vi "Test one or two lift motors.vi"(10 "Direction 2":enum16{"Stop", "Up", "Down"}(ring), 11 "Direction":enum16{"Stop", "Up", "Down"}(ring)) -> ()   [LabVIEW 2014]
uses:
  <vilib>/Rock Robotics/SystemInterfaces/DIO/FPGA_DIOPWMChannel.ctl
  <vilib>/Rock Robotics/WPI/MotorControl/WPI_MotorControlOpen Talon.vi
panel:
  in  "Mode 2":enum8{"Start", "Run", "Finish"}(ring)
  in  "Down Speed 2":dbl=-0.2 format="%#_13g"
  in  "Up Speed 2":dbl=0.3 format="%#_13g"
  in  "Motor one or two":bool
  in  "Mode":enum8{"Start", "Run", "Finish"}(ring)
  in  "Down Speed":dbl=-0.2 format="%#_13g"
  in  "Up Speed":dbl=0.3 format="%#_13g"
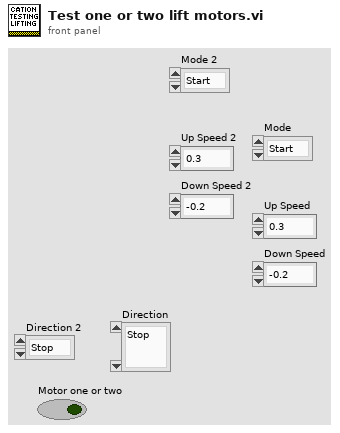
[diagram p1: front panel]
types:
  T1 = typedef "FPGA_DIOPWMChannel.ctl" = enum8{"PWM 0", "PWM 1", "PWM 2", "PWM 3", "PWM 4", "PWM 5", "PWM 6", "PWM 7", "PWM 8", "PWM 9", "PWM MXP 0", "PWM MXP 1", "PWM MXP 2", "PWM MXP 3", "PWM MXP 4", "PWM MXP 5", "PWM MXP 6", "PWM MXP 7", "PWM MXP 8", "PWM MXP 9", "Invalid"}
  T2 = typedef "WPI_MotorControlDeviceRef.ctl" = cluster{"DeviceStatus":errorcluster, "Type":T3, "PWM":cluster{"Controller":T4, "PWM Channel":T1, "DeadBand":T5}, "CAN":cluster{"Device Number":u8, "Control Mode":T6, "Semaphore":T7, "Max Vout":dbl, "TalonSRX Control Mode":T8}, "Invert":bool, "TransformRef":T9, "InvTransformRef":T9}
  T3 = typedef "WPI_MotorControlType.ctl" = enum16{"PWM", "CAN", "CANTalonSRX"}
  T4 = typedef "FPGA_TypedefDigitalModule.ctl" = enum16{"Controller 1"}
  T5 = typedef "WPI_PWMDeadband.ctl" = cluster{"Name":string, "maxPositivePwm":i32, "minPositivePwm":i32, "centerPwm":i32, "maxNegativePwm":i32, "minNegativePwm":i32, "angularRange":u16}
  T6 = typedef "WPI_CANJaguar_ControlMode.ctl" = enum8{"Percent VBus", "Current", "Speed", "Position", "Voltage"}
  T7 = typedef "Semaphore RefNum" = refnum<k1>
  T8 = typedef "WPI_CANTalonSRX_APIControlMode.ctl" = enum8{"Percent VBus", "Speed", "Position", "Slave", "Unchanged / Invalid"}
  T9 = typedef "WPI_PWMTransform_ConPane.ctl" = refnum<vi>
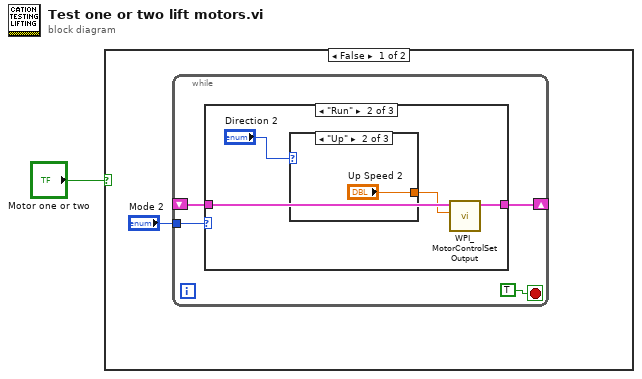
[diagram p0: block diagram]
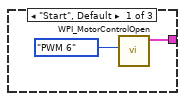
[diagram p2: hidden frame]
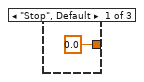
[diagram p3: hidden frame]
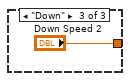
[diagram p4: hidden frame]
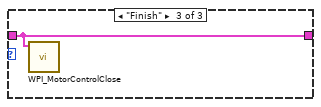
[diagram p5: hidden frame]
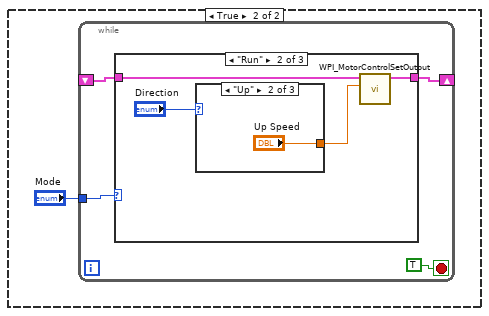
[diagram p6: hidden frame]
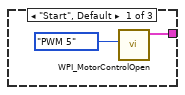
[diagram p7: hidden frame]
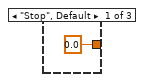
[diagram p8: hidden frame]
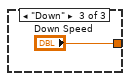
[diagram p9: hidden frame]
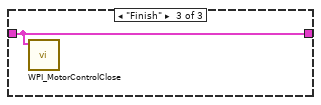
[diagram p10: hidden frame]
diagram:
  n1 = case shown="False" "Motor one or two" {
    frame False {
      n2 = while {
        tunnel: "Mode 2" -> [w5]
        shift-right: [w4] -> _
        shift-left: _ -> [w3]
        stop <- TRUE stop-if-true
        n3 = case shown="\"Run\"" w5 {
          tunnel: [w7 w12 w16] -> w4
          tunnel: w3 -> [_ w11 w16]
          frame "Start", Default {
            n4 = call-poly <vilib>:"WPI_MotorControlOpen.vi"("PWM Channel"=FPGA_DIOPWMChannel."PWM 6") -> ("MotorControlDeviceRef"=w7:T2)  [unwired: 9 in, 1 out]
          }
          frame "Run" {
            n5 = case shown="\"Up\"" "Direction 2" {
              tunnel: [0.0 ("downSpeed") "Up Speed 2" "Down Speed 2"] -> w9
              frame "Stop", Default {
              }
              frame "Up" {
              }
              frame "Down" {
              }
            }
            n6 = call <vilib>:"WPI_MotorControlSetOutput.vi"("Output"=w9, "MotorControlDevRef"=w11) -> ("MotorControlDevRef"=w12:T2)  [unwired: 7 in, 2 out]
          }
          frame "Finish" {
            n7 = call <vilib>:"WPI_MotorControlClose.vi"("MotorControlDevRef"=w16) -> ()  [unwired: 10 in, 1 out]
          }
        }
      }
    }
    frame True {
      n8 = while {
        tunnel: "Mode" -> [w20]
        shift-right: [w19] -> _
        shift-left: _ -> [w18]
        stop <- TRUE stop-if-true
        n9 = case shown="\"Run\"" w20 {
          tunnel: [w22 w26 w31] -> w19
          tunnel: w18 -> [_ w27 w31]
          frame "Start", Default {
            n10 = call-poly <vilib>:"WPI_MotorControlOpen.vi"("PWM Channel"=FPGA_DIOPWMChannel."PWM 5") -> ("MotorControlDeviceRef"=w22:T2)  [unwired: 9 in, 1 out]
          }
          frame "Run" {
            n11 = case shown="\"Up\"" "Direction" {
              tunnel: [0.0 ("downSpeed") "Up Speed" "Down Speed"] -> w24
              frame "Stop", Default {
              }
              frame "Up" {
              }
              frame "Down" {
              }
            }
            n12 = call <vilib>:"WPI_MotorControlSetOutput.vi"("Output"=w24, "MotorControlDevRef"=w27) -> ("MotorControlDevRef"=w26:T2)  [unwired: 7 in, 2 out]
          }
          frame "Finish" {
            n13 = call <vilib>:"WPI_MotorControlClose.vi"("MotorControlDevRef"=w31) -> ()  [unwired: 10 in, 1 out]
          }
        }
      }
    }
  }
